vi "clicked_trajectory.vi"(0 "ScanModeTS090821Circular2D in":refnum<class "ImagingModeTS090821Circular2D.lvclass">, 1 "clicked points":i32[][](array[numeric]), 2 "Numeric":i32, 3 "circular trajectory":bool=TRUE, 7 "error in (no error)":errorcluster) -> (20 "ScanModeTS090821Circular2D out":refnum<class "ImagingModeTS090821Circular2D.lvclass">, 27 "error out":errorcluster)   [LabVIEW 2010, in "ImagingModeTS090821Circular2D.lvclass"]
uses:
  ImagingModeTS090821Circular2D.lvclass
  ImagingModeTS090821Circular2D.lvclass/ImagingModeTS090821Circular2D.ctl
  common/classes/Image/Image/Image.lvclass
  <vilib>/express/express arith-compare/Formula/XNode/ExpressFormulaBlockNode.xnode
  <vilib>/Analysis/BLAS.llb/dnrm2 - Vector 2-Norm (DBL).vi
  <vilib>/Analysis/baseanly.llb/Real Dot Product.vi
  <vilib>/Analysis/NI_AALBase.lvlib
  <vilib>/Analysis/NI_AALBLAS.lvlib
panel:
  out "rotation angle atan2":dbl
  out "x y centering":dbl[](array[numeric])
  out "b amplitude":dbl
  out "a amplitude":dbl
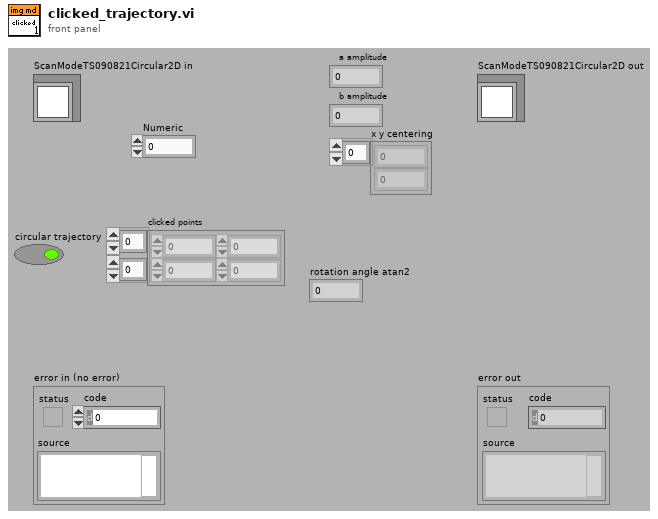
[diagram p1: front panel]
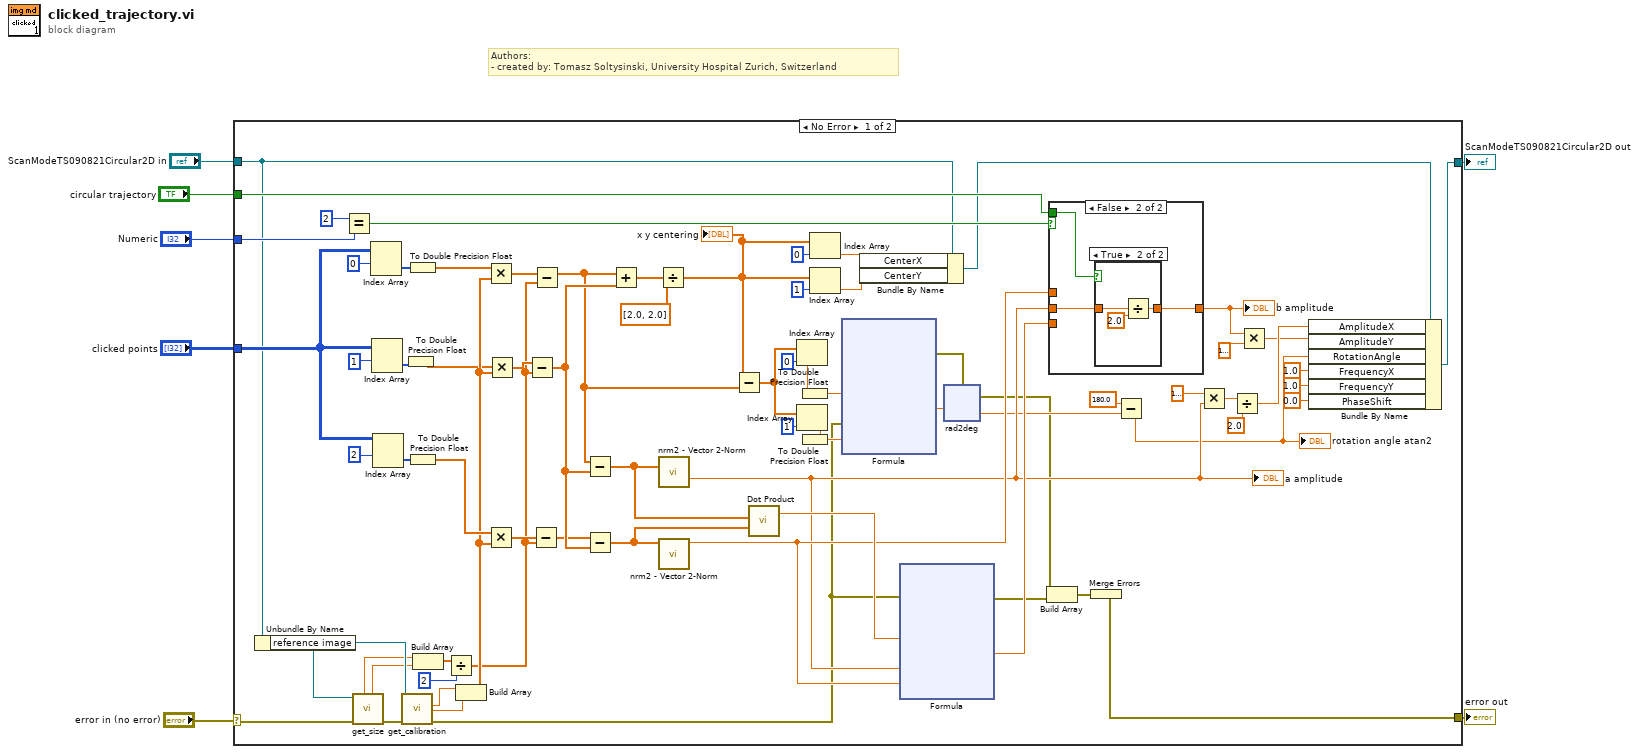
[diagram p0: block diagram]
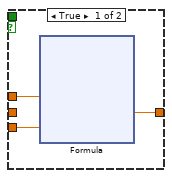
[diagram p2: hidden frame]
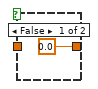
[diagram p3: hidden frame]
diagram:
  # "Authors: \n- created by: Tomasz Soltysinski, University Hospital Zurich, Switzerland"
  n1 = case shown="No Error" "error in (no error)" {
    selector: "error in (no error)" -> [w21 w133]
    tunnel: [w56 w133] -> w6
    tunnel: [w58 w132] -> w4
    tunnel: "ScanModeTS090821Circular2D in" -> [w25 w132]
    tunnel: "clicked points" -> [w37 _]
    tunnel: "Numeric" -> [w74 _]
    tunnel: "circular trajectory" -> [w76 _]
    frame No Error {
      n2 = Unbundle By Name(w25) -> ("reference image"=w19:refnum<class "Image.lvclass">)
      n3 = Equal?(x=2, y=w74) -> (x = y?=w80:bool)
      n4 = call-dynamic "get_size.vi"("error in (no error)"=w21, "Image in"=w19) -> ("error out"=w20:errorcluster, "physical size y"=w17:dbl, "physical size x"=w18:dbl)  [unwired: 2 in, 5 out]
      n5 = Index Array(array=w37, index (row)=0 ("disabled index (col)")) -> (element=w36:i32[])  [unwired: 1 in]
      n6 = Index Array(array=w37, index (row)=1 ("disabled index (col)")) -> (element=w35:i32[])  [unwired: 1 in]
      n7 = Index Array(array=w37, index (row)=2 ("disabled index (col)")) -> (element=w34:i32[])  [unwired: 1 in]
      n8 = call "get_calibration.vi"("error in (no error)"=w20, "Image.lvclass in"=w19) -> ("error out"=w24:errorcluster, "y"=w22:dbl, "x"=w23:dbl)  [unwired: 4 in, 3 out]
      n9 = To Double Precision Float(number=w35) -> (double precision float=w28:dbl[])
      n10 = To Double Precision Float(number=w36) -> (double precision float=w27:dbl[])
      n11 = To Double Precision Float(number=w34) -> (double precision float=w30:dbl[])
      n12 = Build Array(w18, w17) -> (w10:dbl[])
      n13 = Divide(x=w10, y=2 ("physical size y")) -> (x/y=w9:dbl[])
      n14 = Build Array(w23, w22) -> (w29:dbl[])
      n15 = Multiply(x=w27, y=w29) -> (x*y=w14:dbl[])
      n16 = Multiply(x=w30, y=w29) -> (x*y=w12:dbl[])
      n17 = Multiply(x=w28, y=w29) -> (x*y=w16:dbl[])
      n18 = Subtract(x=w16, y=w9) -> (x-y=w15:dbl[])
      n19 = Subtract(x=w12, y=w9) -> (x-y=w11:dbl[])
      n20 = Subtract(x=w14, y=w9) -> (x-y=w13:dbl[])
      n21 = Subtract(x=w13, y=w15) -> (x-y=w32:dbl[])
      n22 = Subtract(x=w11, y=w15) -> (x-y=w31:dbl[])
      n23 = Add(x=w13, y=w15) -> (x+y=w33:dbl[])
      n24 = Divide(x=w33, y=dbl[] [2.0, 2.0]) -> (x/y=w26:dbl[])
      "x y centering" <- w26
      n25 = call-poly <vilib>:"nrm2 - Vector 2-Norm.vi"("x"=w32) -> ("dnrm2"=w60:dbl)  [unwired: 9 in, 1 out]
      "a amplitude" <- w60
      n26 = call-poly <vilib>:"nrm2 - Vector 2-Norm.vi"("x"=w31) -> ("dnrm2"=w78:dbl)  [unwired: 9 in, 1 out]
      n27 = Subtract(x=w26, y=w13) -> (x-y=w53:dbl[])
      n28 = call-poly <vilib>:"Dot Product.vi"("Y Vector"=w31, "X Vector"=w32) -> ("X * Y"=w79:dbl)  [unwired: 1 out]
      n29 = Index Array(array=w53, index=0) -> (element=w52:dbl)
      n30 = Index Array(array=w53, index=1) -> (element=w50:dbl)
      n31 = To Double Precision Float(number=w52) -> (double precision float=w51:dbl)
      n32 = To Double Precision Float(number=w50) -> (double precision float=w49:dbl)
      n33 = Index Array(array=w26, index=0 ("disabled index (col)")) -> (element=w63:dbl)
      n34 = Index Array(array=w26, index=1 ("disabled index (col)")) -> (element=w61:dbl)
      n35 = xnode "Formula"("x"=w51, "error in (no error)"=w24, "y"=w49) -> ("Result"=w47:dbl, "error out"=w45:errorcluster)
      n36 = Bundle By Name(cluster=w25, "CenterX"=w63, "CenterY"=w61) -> (w59:refnum<class "ImagingModeTS090821Circular2D.lvclass">)
      n37 = xnode "Formula"("dot_u_v"=w79, "u"=w60, "v"=w78, "error in (no error)"=w24) -> ("Result"=w77:dbl, "error out"=w43:errorcluster)
      n38 = xnode "rad2deg"("alfa"=w47, "error in (no error)"=w45) -> ("Result"=w46:dbl, "error out"=w44:errorcluster)
      n39 = Build Array(w44, w43) -> (w57:errorcluster[])
      n40 = case shown="False" w80 {
        tunnel: w78 -> [w114 _]
        tunnel: w77 -> [w113 _]
        tunnel: [w112 w127] -> w72
        tunnel: w76 -> [_ w126]
        tunnel: w60 -> [_ w125]
        frame True {
          n41 = xnode "Formula"("a"=w114, "alfa"=w113) -> ("Result"=w112:dbl)  [unwired: 1 in, 1 out]
        }
        frame False, Default {
          n42 = case shown="True" w126 {
            tunnel: [0.0 ("Result") w129] -> w127
            tunnel: w125 -> [_ w130]
            frame False {
            }
            frame True {
              n43 = Divide(x=w130, y=2.0) -> (x/y=w129:dbl)
            }
          }
        }
      }
      "b amplitude" <- w72
      n44 = Merge Errors(w57) -> (w56:errorcluster)
      n45 = Subtract(x=180.0 ("y"), y=w46) -> (x-y=w38:dbl)
      "rotation angle atan2" <- w38
      n46 = Multiply(x=dbl[unit] 1e-06 ("dimension size"), y=w60) -> (x*y=w68:dbl[unit])
      n47 = Divide(x=w68, y=2.0) -> (x/y=w66:dbl[unit])
      n48 = Multiply(x=w72, y=dbl[unit] 1e-06 ("dimension size")) -> (x*y=w39:dbl[unit])
      n49 = Bundle By Name(cluster=w59, "AmplitudeX"=w66, "AmplitudeY"=w39, "RotationAngle"=w38, "FrequencyX"=1.0 ("settings.x frequency"), "FrequencyY"=1.0 ("settings.y frequency"), "PhaseShift"=0.0 ("settings.phase shift")) -> (w58:refnum<class "ImagingModeTS090821Circular2D.lvclass">)
    }
    frame Error {
    }
  }
  "error out" <- w6
  "ScanModeTS090821Circular2D out" <- w4
